vi "Car Go Left.vi"(9 "m array":i16[][](array[numeric]), 10 "Numeric":i32, 11 "Input in":i32[][](array[numeric])) -> (2 "move or not":bool, 3 "Input out":i32[][](array[numeric]))   [LabVIEW 2021]
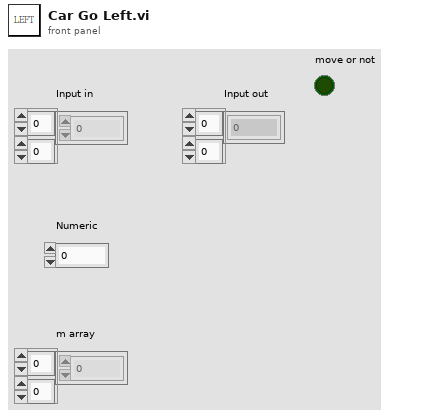
[diagram p1: front panel]
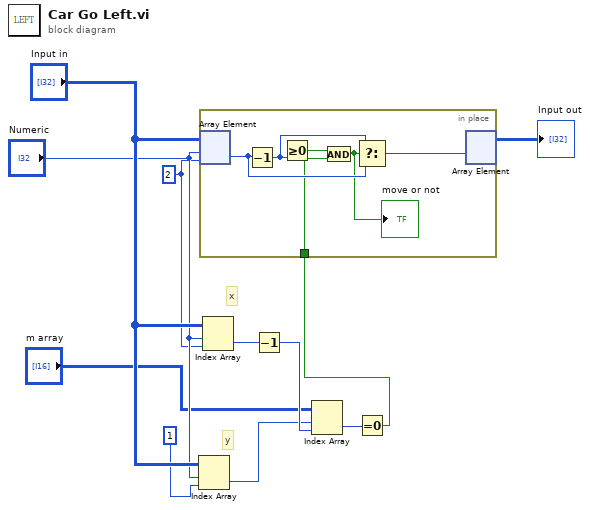
[diagram p0: block diagram]
diagram:
  w3 = 2
  # "y"
  # "x"
  n1 = Index Array(array="Input in", index (row)="Numeric", index (col)=1) -> (element=w6:i32)
  n2 = Index Array(array="Input in", index (row)="Numeric", index (col)=w3) -> (element=w10:i32)
  n3 = Decrement(x=w10) -> (x-1=w8:i32)
  n4 = Index Array(array="m array", index (row)=w6, index (col)=w8) -> (element=w9:i16)
  n5 = Equal To 0?(x=w9) -> (x = 0?=w11:bool)
  n6 = in-place {
    in-place-border: w11 -> [w12]
    n7 = in-place-array #1("Input in", "Numeric", w3) -> (w14:i32)
    n8 = Decrement(x=w14) -> (x-1=w15:i32)
    n9 = Greater Or Equal To 0?(x=w15) -> (x >= 0?=w17:bool)
    n10 = And(x=w17, y=w12) -> (x .and. y?=w13:bool)
    "move or not" <- w13
    n11 = Select(t=w15, s=w13, f=w14) -> (s? t:f=w16:i32)
    n12 = in-place-array #1(w16) -> (→"Input out":i32[][])  [unwired: 2 out]
  }
